vi "Finish Scan.vi"(8 "error in (no error)":errorcluster, 11 "Scanner in":refnum<class "Scanner.lvclass">) -> (0 "error out":errorcluster, 3 "Scanner out":refnum<class "Scanner.lvclass">)   [LabVIEW 2023, in "Scanner.lvclass"]
doc: "(Dynamic) Perform any cleanup after the last step. Restore the instrument to its initial pre-scan state if \"Return to Start\" is true."
uses:
  Scanner.lvclass
  Scanner.lvclass/Scanner.ctl
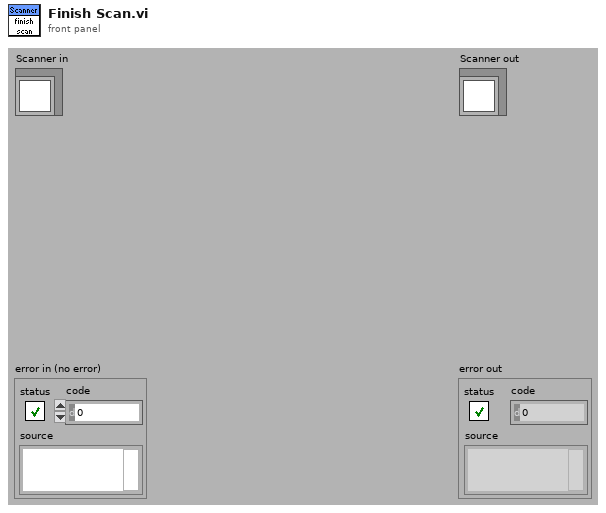
[diagram p1: front panel]
types:
  T1 = typedef "Scanner.lvclass/Range.ctl" = cluster{"xi":dbl, "xf":dbl, "dx":dbl, "Return to...?":bool, "Return to":dbl}
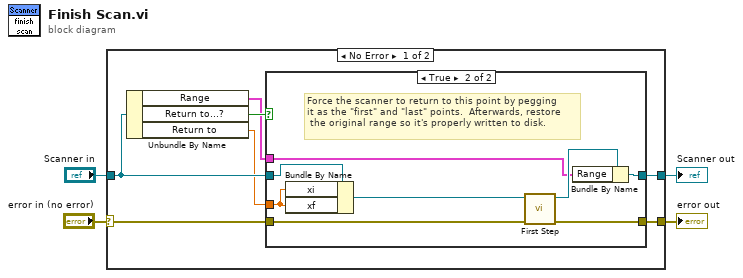
[diagram p0: block diagram]
diagram:
  n1 = case shown="No Error" "error in (no error)" {
    selector: "error in (no error)" -> [w8 w23]
    tunnel: [w7 w23] -> w3
    tunnel: [w9 w22] -> w1
    tunnel: "Scanner in" -> [w10 w22]
    frame No Error {
      n2 = Unbundle By Name(w10) -> ("Range"=w5:T1, "Return to...?"=w11:bool, "Return to"=w6:dbl)
      n3 = case shown="True" w11 {
        tunnel: w8 -> [w12 w14]
        tunnel: w10 -> [w13 w21]
        tunnel: [w13 w16] -> w9
        tunnel: [w12 w15] -> w7
        tunnel: w6 -> [_ w20]
        tunnel: w5 -> [_ w17]
        frame False {
        }
        frame True {
          # "Force the scanner to return to this point by pegging\nit as the \"first\" and \"last\" points.  Afterwards, restore\n the original range so it's properly written to disk."
          n4 = Bundle By Name(cluster=w21, "xi"=w20, "xf"=w20) -> (w19:refnum<class "Scanner.lvclass">)
          n5 = call-dynamic "First Step.vi"("error in (no error)"=w14, "Scanner.lvclass in"=w19) -> ("error out"=w15:errorcluster, "Scanner.lvclass out"=w18:refnum<class "Scanner.lvclass">)  [unwired: 7 in, 1 out]
          n6 = Bundle By Name(cluster=w18, "Range"=w17) -> (w16:refnum<class "Scanner.lvclass">)
        }
      }
    }
    frame Error {
    }
  }
  "error out" <- w3
  "Scanner out" <- w1
